vi "Probability Density.vi"() -> ()   [LabVIEW 2023]
doc: "Generates a probability density function and a probability distribution function using the Histogram, Integral x(t), and Derivative x(t) VIs. The input signal is Gaussian or uniform noise. You can also add two additional variables and test the Central Limit Theorem."
uses:
  <vilib>/gmath/statdist.llb/Normal Random.vi
  <vilib>/gmath/statdist.llb/Uniform Random.vi
  <vilib>/Analysis/NI_AALPro.lvlib
  <vilib>/gmath/NI_Gmath.lvlib
panel:
  in  "Variable 1":u16(ring)=2 items=["None", "Gaussian", "Uniform"]
  in  "Variable 3":u16(ring) items=["None", "Gaussian", "Uniform"]
  in  "Variable 2":u16(ring) items=["None", "Gaussian", "Uniform"]
  out "Histogram Graph":cluster{dbl[], "Axis":dbl[]}(graph)
  in  "Stop":bool
  out "Waveform Graph":dbl[](graph)
  in  "Probability Samples":i32=50
  in  "# of iterations":i32(slide)=500 scale=1.0..1000.0
  in  "Samples/iteration":i32=5000
  out "Probability Density Function (PDF)":cluster{"Ramp Pattern":dbl[], dbl[]}(graph)
  out "Cumulative Density Function (CDF)":cluster{"Ramp Pattern":dbl[], dbl[]}(graph)
  # "Overview: Generates a probability density function (PDF) and a cumulative probability density function (CDF) using the General Histogram VI, Integral x(t) VI, and Derivative x(t) VI.\nRequirements: LabVIEW Full Development System\nInstructions:\n1. Run the VI and set Variable 1 as \"Uniform\" or \"Gaussian\" and verify the Histogram, PDF, and CDF being generated.\n2. Change Variable 1 to \"Uniform\" and Variable 2 to \"Uniform\". The PDF formed will resemble a 'triangular' distribution. If you change Variable 3 to \"Uniform\", this will start to resemble a gaussian distribution, as defined by the Central Limit Theorem.\n3. Change the histogram parameters and verify that this would make the evaluation of the PDF and CDF worse.\n4. Click Stop to stop the VI."
  # "Signal Generation"
  # "Histogram Parameters"
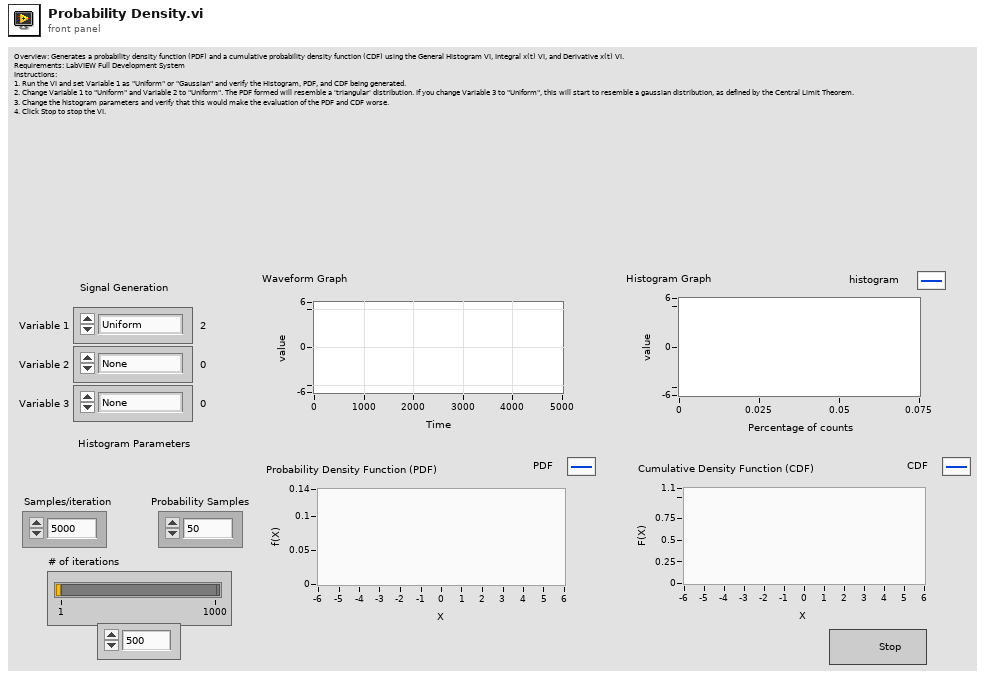
[diagram p1: front panel]
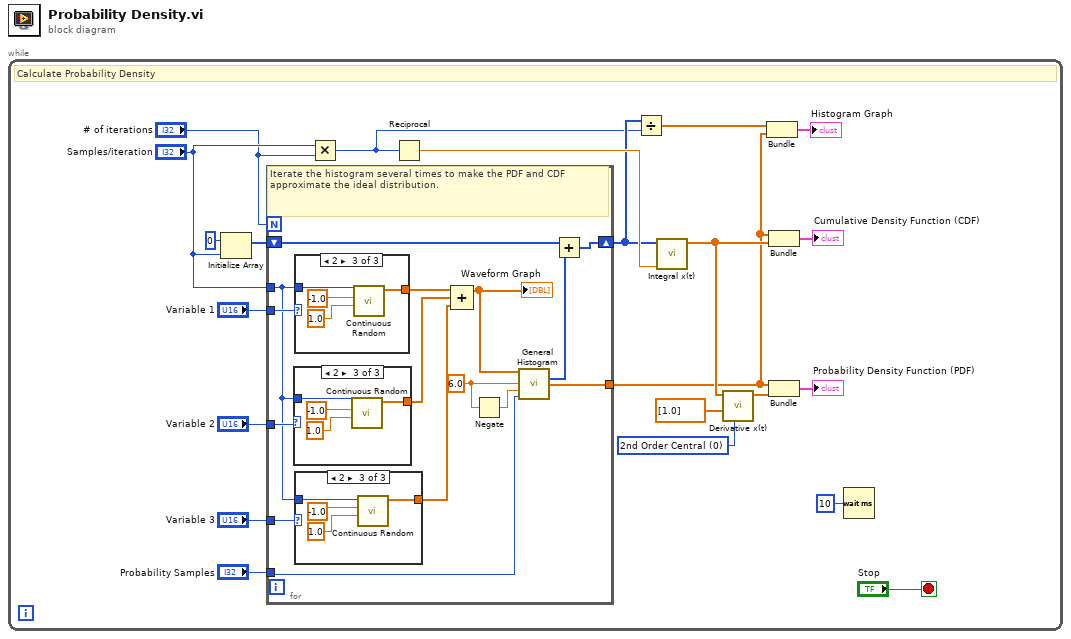
[diagram p0: block diagram]
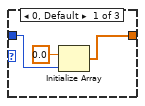
[diagram p2: hidden frame]
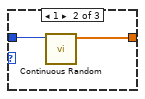
[diagram p3: hidden frame]
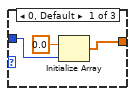
[diagram p4: hidden frame]
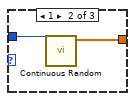
[diagram p5: hidden frame]
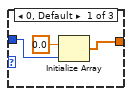
[diagram p6: hidden frame]
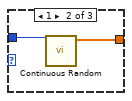
[diagram p7: hidden frame]
diagram:
  n1 = while {
    stop <- "Stop" stop-if-true
    w12 = u16 0 items=["2nd Order Central", "4th Order Central", "Forward", "Backward"] ("method")
    # "Calculate Probability Density"
    n2 = Initialize Array(0, "Samples/iteration") -> (w22:i32[])
    n3 = for {
      N: "# of iterations" -> [_]
      shift-right: [w35] -> w10
      shift-left: w22 -> [w36]
      tunnel: "Samples/iteration" -> [w28]
      tunnel: "Probability Samples" -> [w37]
      tunnel: [w34] -> w9
      tunnel: "Variable 2" -> [w30]
      tunnel: "Variable 1" -> [w31]
      tunnel: "Variable 3" -> [w29]
      w27 = 6.0 ("max")
      # "Iterate the histogram several times to make the PDF and CDF approximate the ideal distribution."
      n4 = case shown="2" w30 {
        tunnel: w28 -> [w48 w51 w55]
        tunnel: [w49 w50 w54] -> w24
        frame 0, Default {
          n5 = Initialize Array(0.0 ("element"), w48) -> (w49:dbl[])
        }
        frame 1 {
          n6 = call-poly <vilib>:"Continuous Random.vi"("samples"=w51) -> ("normal random data"=w50:dbl[])  [unwired: 9 in, 1 out]
        }
        frame 2 {
          n7 = call-poly <vilib>:"Continuous Random.vi"("xmax"=1.0, "xmin"=-1.0, "samples"=w55) -> ("uniform random data"=w54:dbl[])  [unwired: 7 in, 1 out]
        }
      }
      n8 = case shown="2" w31 {
        tunnel: w28 -> [w57 w60 w64]
        tunnel: [w58 w59 w63] -> w23
        frame 0, Default {
          n9 = Initialize Array(0.0 ("element"), w57) -> (w58:dbl[])
        }
        frame 1 {
          n10 = call-poly <vilib>:"Continuous Random.vi"("samples"=w60) -> ("normal random data"=w59:dbl[])  [unwired: 9 in, 1 out]
        }
        frame 2 {
          n11 = call-poly <vilib>:"Continuous Random.vi"("xmax"=1.0, "xmin"=-1.0, "samples"=w64) -> ("uniform random data"=w63:dbl[])  [unwired: 7 in, 1 out]
        }
      }
      n12 = case shown="2" w29 {
        tunnel: w28 -> [w39 w42 w46]
        tunnel: [w40 w41 w45] -> w25
        frame 0, Default {
          n13 = Initialize Array(0.0 ("element"), w39) -> (w40:dbl[])
        }
        frame 1 {
          n14 = call-poly <vilib>:"Continuous Random.vi"("samples"=w42) -> ("normal random data"=w41:dbl[])  [unwired: 9 in, 1 out]
        }
        frame 2 {
          n15 = call-poly <vilib>:"Continuous Random.vi"("xmax"=1.0, "xmin"=-1.0, "samples"=w46) -> ("uniform random data"=w45:dbl[])  [unwired: 7 in, 1 out]
        }
      }
      n16 = Compound Arithmetic op=ADD(w23, w24, w25) -> (w32:dbl[])
      "Waveform Graph" <- w32
      n17 = Negate(x=w27) -> (-x=w26:dbl)
      n18 = call <vilib>:"General Histogram.vi"("X"=w32, "max"=w27, "min"=w26, "# bins"=w37) -> ("Histogram"=w33:i32[], "Axis"=w34:dbl[])  [unwired: 7 in, 3 out]
      n19 = Add(x=w36, y=w33) -> (x+y=w35:i32[])
    }
    n20 = Multiply(x="Samples/iteration", y="# of iterations") -> (x*y=w2:i32)
    n21 = Reciprocal(x=w2) -> (1/x=w15:dbl)
    n22 = Divide(x=w10, y=w2) -> (x/y=w4:dbl[])
    n23 = call <vilib>:"Integral x(t).vi"("dt"=w15, "X"=w10) -> ("Integral X"=w19:dbl[])  [unwired: 8 in, 1 out]
    n24 = call <vilib>:"Derivative x(t).vi"("method"=w12, "Final Condition"=dbl[] [1.0] ("final condition"), "X"=w19) -> ("dX/dt"=w18:dbl[])  [unwired: 7 in, 1 out]
    n25 = Bundle(w4, "Axis"=w9) -> (→"Histogram Graph":cluster{dbl[], "Axis":dbl[]})  [unwired: 1 in]
    n26 = Bundle("Axis"=w9, "Integral X"=w19) -> (→"Cumulative Density Function (CDF)":cluster{"Axis":dbl[], "Integral X":dbl[]})  [unwired: 1 in]
    n27 = Bundle("Axis"=w9, "dX/dt"=w18) -> (→"Probability Density Function (PDF)":cluster{"Axis":dbl[], "dX/dt":dbl[]})  [unwired: 1 in]
    n28 = Wait (ms)(milliseconds to wait=u32 10) -> ()  [unwired: 1 out]
  }
